vi "AVS_Get-Interpolated-T.vi"(9 "# of Data Points":dbl, 10 "Calibration Datapoints":dbl[][](array[numeric])=[[3.4398, 6.127], [3.4398, 6.122], [3.4398, 5.876], [0.0, 0.0], [0.0, 0.0], [0.0, 0.0], [0.0, 0.0], [0.0, 0.0], [0.0, 0.0], [0.0, 0.0], [0.0, 0.0], [0.0, 0.0], [0.0, 0.0], [0.0, 0.0], [0.0, 0.0], [0.0, 0.0], [0.0, 0.0], [0.0, 0.0], [0.0, 0.0], [0.0, 0.0], [0.0, 0.0], [0.0, 0.0], [0.0, 0.0], [0.0, 0.0], [0.0, 0.0], [0.0, 0.0], [0.0, 0.0], [0.0, 0.0], [0.0, 0.0], [0.0, 0.0], [0.0, 0.0], [0.0, 0.0], [0.0, 0.0], [0.0, 0.0], [0.0, 0.0], [0.0, 0.0], [0.0, 0.0], [0.0, 0.0], [0.0, 0.0], [0.0, 0.0], [0.0, 0.0], [0.0, 0.0], [0.0, 0.0], [0.0, 0.0], [0.0, 0.0], [0.0, 0.0], [0.0, 0.0], [0.0, 0.0], [0.0, 0.0], [0.0, 0.0], [0.0, 0.0], [0.0, 0.0], [0.0, 0.0], [0.0, 0.0], [0.0, 0.0], [0.0, 0.0], [0.0, 0.0], [0.0, 0.0], [0.0, 0.0], [0.0, 0.0], [0.0, 0.0], [0.0, 0.0], [0.0, 0.0], [0.0, 0.0], [0.0, 0.0], [0.0, 0.0], [0.0, 0.0], [0.0, 0.0], [0.0, 0.0], [0.0, 0.0], [0.0, 0.0], [0.0, 0.0], [0.0, 0.0], [0.0, 0.0], [0.0, 0.0], [0.0, 0.0], [0.0, 0.0], [0.0, 0.0], [0.0, 0.0], [0.0, 0.0], [0.0, 0.0], [0.0, 0.0], [0.0, 0.0], [0.0, 0.0], [0.0, 0.0], [0.0, 0.0], [0.0, 0.0], [0.0, 0.0], [0.0, 0.0], [0.0, 0.0], [0.0, 0.0], [0.0, 0.0], [0.0, 0.0], [0.0, 0.0], [0.0, 0.0], [0.0, 0.0], [0.0, 0.0], [0.0, 0.0], [0.0, 0.0], [0.0, 0.0], [0.0, 0.0], [0.0, 0.0], [0.0, 0.0], [0.0, 0.0], [0.0, 0.0], [0.0, 0.0], [0.0, 0.0], [0.0, 0.0], [0.0, 0.0], [0.0, 0.0], [0.0, 0.0], [0.0, 0.0], [0.0, 0.0], [0.0, 0.0], [0.0, 0.0], [0.0, 0.0], [0.0, 0.0], [0.0, 0.0], [0.0, 0.0], [0.0, 0.0], [0.0, 0.0], [0.0, 0.0], [0.0, 0.0], [0.0, 0.0], [0.0, 0.0], [0.0, 0.0], [0.0, 0.0], [0.0, 0.0], [0.0, 0.0], [0.0, 0.0], [0.0, 0.0], [0.0, 0.0], [0.0, 0.0], [0.0, 0.0], [0.0, 0.0], [0.0, 0.0], [0.0, 0.0]], 11 "Resistance value":dbl) -> (3 "Interpolated Termperature scalar":dbl)   [LabVIEW 2019]
panel:
  out "Log Resistance":dbl
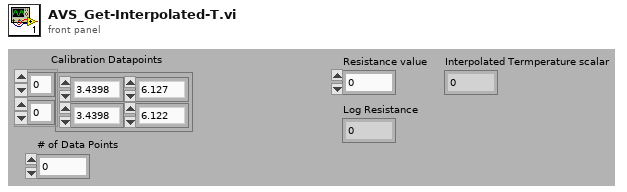
[diagram p1: front panel]
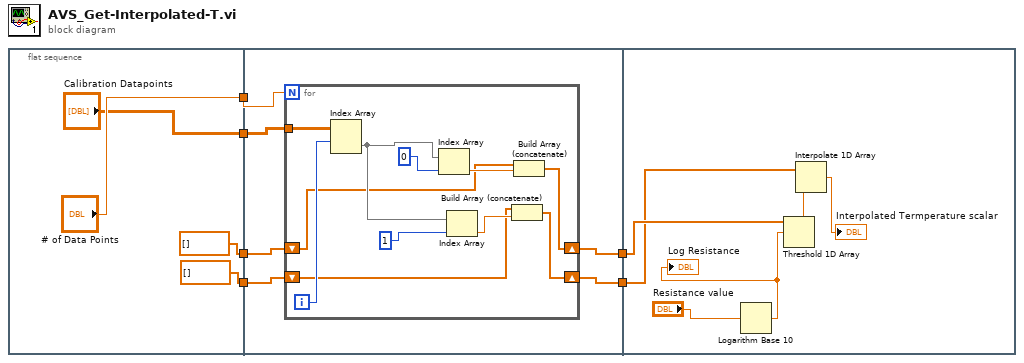
[diagram p0: block diagram]
diagram:
  n1 = flat-sequence {
    tunnel: ["Calibration Datapoints"] -> w6
    tunnel: ["# of Data Points"] -> w5
    tunnel: [dbl[] []] -> w4
    tunnel: [dbl[] []] -> w3
    tunnel: w6 -> [w11]
    tunnel: w5 -> [w16]
    tunnel: w4 -> [w15]
    tunnel: w3 -> [w14]
    tunnel: [w13] -> w2
    tunnel: [w12] -> w1
    tunnel: w2 -> [w29]
    tunnel: w1 -> [w28]
    frame #0 {
    }
    frame #1 {
      n2 = for {
        N: w16 -> [_]
        shift-right: [w19] -> w13
        shift-left: w15 -> [w21]
        shift-right: [w18] -> w12
        shift-left: w14 -> [w20]
        tunnel: w11 -> [w17]
        i -> [w25]
        n3 = Index Array(array=w17, index (row)=w25) -> (element=w24:dbl[])  [unwired: 1 in]
        n4 = Index Array(array=w24, index=0) -> (element=w23:dbl)
        n5 = Index Array(array=w24, index=1) -> (element=w22:dbl)
        n6 = Build Array (concatenate)(w20, w22) -> (w18:dbl[])
        n7 = Build Array (concatenate)(w21, w23) -> (w19:dbl[])
      }
    }
    frame #2 {
      n8 = Logarithm Base 10(1:"Resistance value") -> (0:w31:dbl)
      "Log Resistance" <- w31
      n9 = Threshold 1D Array(2:w31, 3:w29) -> (0:w33:dbl)  [unwired: 1 in]
      n10 = Interpolate 1D Array(1:w33, 2:w28) -> (0:→"Interpolated Termperature scalar":dbl)
    }
  }
